vi "ge_GetGrpChans_NGrp.vi"(10 "Chassis Name":tag, 11 "HS Groups":T2[](array[typedef])) -> (1 "Num of Chans":i32, 2 "Multi Rate Mods in Grp":T1, 3 "All Rate Chans":string[](array[string]))   [LabVIEW 2011]
uses:
  Custom Ctrls/Master Cfg/ge_ChannelGroup.ctl
  Custom Ctrls/ge_MeasType.ctl
  Classes/Channel/Channel.lvclass
  Custom Ctrls Bld/ge_MultiRateMods.ctl
  Classes/Channel/Read ChanName.vi
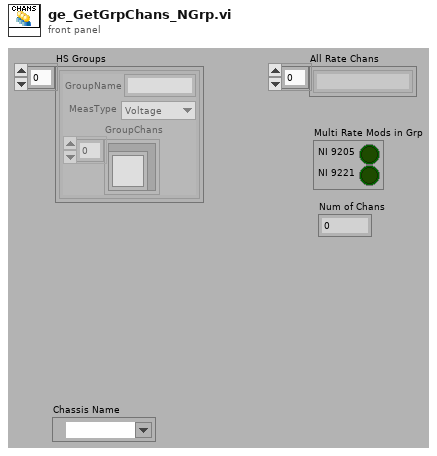
[diagram p1: front panel]
types:
  T1 = typedef "ge_MultiRateMods.ctl" = cluster{"NI 9205":bool, "NI 9221":bool}
  T2 = typedef "ge_ChannelGroup.ctl" = cluster{"GroupName":string, "MeasType":T3, "GroupChans":refnum<class "Channel.lvclass">[]}
  T3 = typedef "ge_MeasType.ctl" = enum16{"Voltage", "Frequency", "Tachometer", "Dynamic", "Thermocouple", "RTD", "Strain", "Current", "Resistance"}
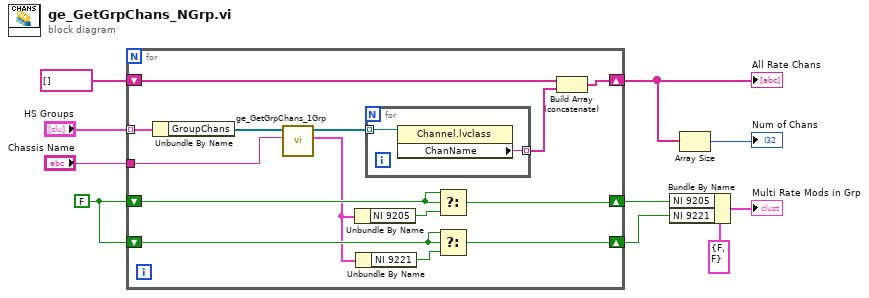
[diagram p0: block diagram]
diagram:
  w10 = FALSE
  n1 = for {
    tunnel: "HS Groups" -> [w12] mode=indexing
    shift-right: [w22] -> w7
    shift-left: w10 -> [w24]
    shift-right: [w19] -> w6
    shift-left: w10 -> [w21]
    shift-right: [w17] -> w2
    shift-left: string[] [] ("Grp Chans") -> [w18]
    tunnel: "Chassis Name" -> [w16]
    n2 = Unbundle By Name(w12) -> ("GroupChans"=w11:refnum<class "Channel.lvclass">[])
    n3 = call "ge_GetGrpChans_1Grp.vi"("Chassis Name"=w16, "GroupChansIn"=w11) -> ("Multi Rate Mods in Grp"=w15:T1, "GroupChansOut"=w14:refnum<class "Channel.lvclass">[])  [unwired: 5 in, 3 out]
    n4 = Unbundle By Name(w15) -> ("NI 9205"=w23:bool)
    n5 = Unbundle By Name(w15) -> ("NI 9221"=w20:bool)
    n6 = for {
      tunnel: w14 -> [w26] mode=indexing
      tunnel: [w25] -> w13 mode=indexing
      n7 = property class="Channel.lvclass"(reference=w26) -> ("ChanName"=w25:string)  [unwired: 1 in, 2 out]
    }
    n8 = Select(t=w24, s=w24, f=w23) -> (s? t:f=w22:bool)
    n9 = Select(t=w21, s=w21, f=w20) -> (s? t:f=w19:bool)
    n10 = Build Array (concatenate)(w18, w13) -> (w17:string[])
  }
  "All Rate Chans" <- w2
  n11 = Bundle By Name(cluster=T1 {"NI 9205"=FALSE, "NI 9221"=FALSE} ("Multi Rate Mods in Grp"), "NI 9205"=w7, "NI 9221"=w6) -> (→"Multi Rate Mods in Grp":T1)
  n12 = Array Size(array=w2) -> (size(s)=→"Num of Chans":i32)
